vi "Do Mutate.vi"(8 "error in":errorcluster, 10 "IGene in":refnum<class "IGene.lvclass">, 11 "Mutator in":refnum<class "Mutator.lvclass">) -> (0 "error out":errorcluster, 2 "IGene out":refnum<class "IGene.lvclass">, 3 "Mutator out":refnum<class "Mutator.lvclass">)   [LabVIEW 2016, in "Mutator.lvclass"]
uses:
  Mutator.lvclass
  IGene/IGene.lvclass
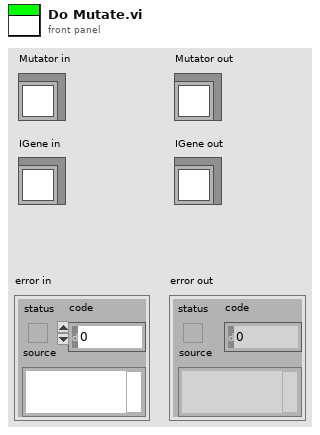
[diagram p1: front panel]
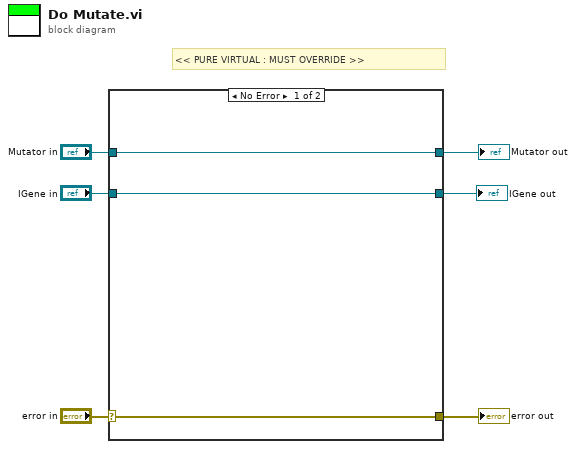
[diagram p0: block diagram]
diagram:
  # "<< PURE VIRTUAL : MUST OVERRIDE >>"
  n1 = case shown="No Error" "error in" {
    selector: "error in" -> [w8 w12]
    tunnel: [w8 w12] -> w5
    tunnel: [w9 w11] -> w3
    tunnel: "Mutator in" -> [w9 w11]
    tunnel: "IGene in" -> [w7 w10]
    tunnel: [w7 w10] -> w1
    frame No Error {
    }
    frame Error {
    }
  }
  "error out" <- w5
  "Mutator out" <- w3
  "IGene out" <- w1
